vi "Write_Single_Reg.vi"(2 "Reg No":u8 format="%x", 3 "Write I2C Address":u8 format="%x", 4 "Reg Value":u16 format="%x", 5 "USB DAQ Address":i32 format="%x") -> (0 "Status String":string="ERROR COMMUNICATING WITH DEVICE")   [LabVIEW 2011]
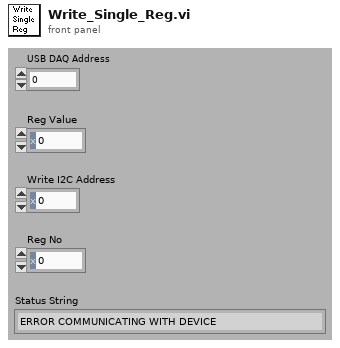
[diagram p1: front panel]
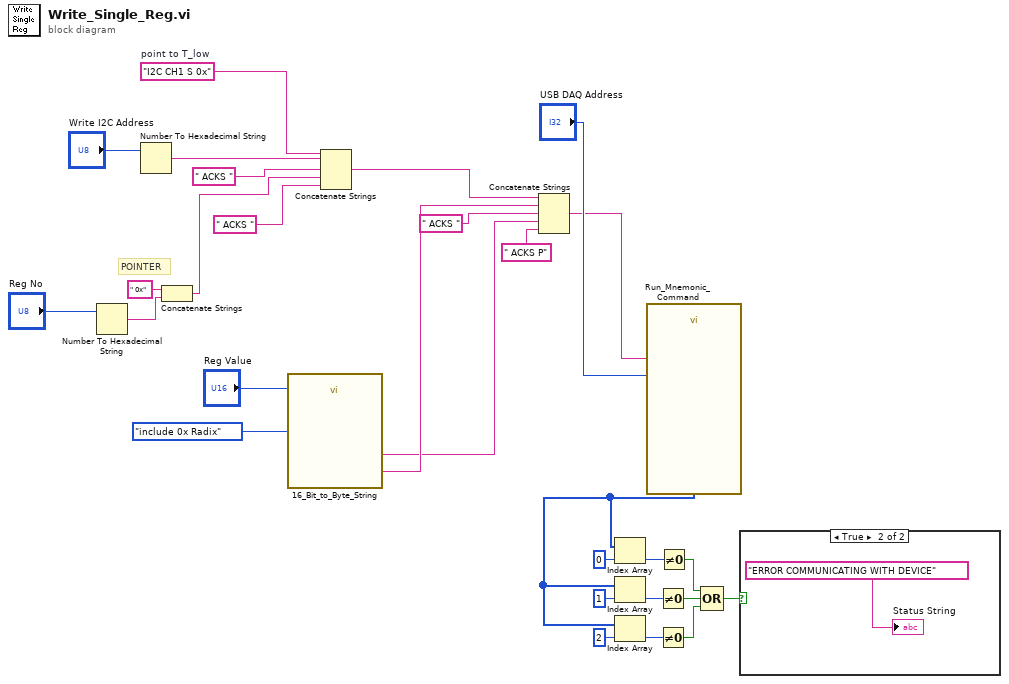
[diagram p0: block diagram]
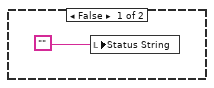
[diagram p2: hidden frame]
diagram:
  w21 = "I2C CH1 S 0x"  # point to T_low
  # "POINTER"
  n1 = Number To Hexadecimal String(2:"Reg No") -> (0:w27:string)  [unwired: 1 in]
  n2 = Number To Hexadecimal String(2:"Write I2C Address") -> (0:w22:string)  [unwired: 1 in]
  n3 = Concatenate Strings(" 0x" ("string"), w27) -> (w26:string)
  n4 = call "16_Bit_to_Byte_String.vi"("Radix Format"=enum32{"include 0x Radix", "No Radix"}."include 0x Radix", "16 bit in"="Reg Value") -> ("LSB OUT"=w12:string, "MSB OUT"=w13:string)
  n5 = Concatenate Strings(w21, w22, " ACKS " ("string"), w26, " ACKS " ("string")) -> (w25:string)
  n6 = Concatenate Strings(w25, w13, " ACKS " ("string"), w12, " ACKS P" ("string")) -> (w16:string)
  n7 = call "Run_Mnemonic_Command.vi"("command string"=w16, "Device address"="USB DAQ Address") -> ("ACKS-array"=w1:u8[])  [unwired: 2 in, 4 out]
  n8 = Index Array(array=w1, index=0) -> (element=w5:u8)
  n9 = Index Array(array=w1, index=1) -> (element=w10:u8)
  n10 = Index Array(array=w1, index=2) -> (element=w7:u8)
  n11 = Not Equal To 0?(x=w10) -> (x != 0?=w6:bool)
  n12 = Not Equal To 0?(x=w7) -> (x != 0?=w8:bool)
  n13 = Not Equal To 0?(x=w5) -> (x != 0?=w9:bool)
  n14 = Compound Arithmetic op=OR(w9, w6, w8) -> (w11:bool)
  n15 = case shown="True" w11 {
    frame False {
      n16 = local write "Status String"("") -> ()
    }
    frame True {
      "Status String" <- "ERROR COMMUNICATING WITH DEVICE"
    }
  }
